vi "Process Dichotomie.vi"(7 "Movable in":refnum<class "Movable.lvclass">, 11 "Collision in":refnum<class "Collision.lvclass">) -> (2 "Coordinates with dichotomie[] out":T1[](array[typedef]), 5 "Dichotomie out":i32=10)   [LabVIEW 2021, in "Collision.lvclass"]
doc: "MIT Licence\nCopyright (c) 2024 David Grollier"
uses:
  Collision.lvclass
  Type Def/Coordinates.ctl
  Game Componants/Game Board Component/Movable/Movable.lvclass
  Game Componants/Game Board/Game Board.lvclass
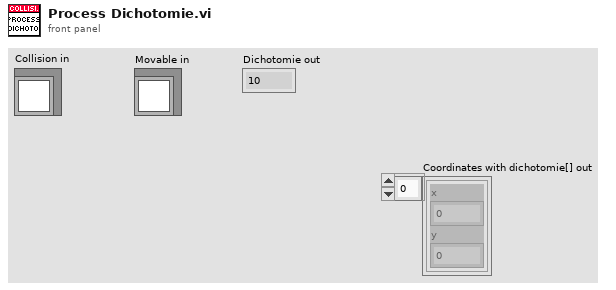
[diagram p1: front panel]
types:
  T1 = typedef "Coordinates.ctl" = cluster{"x":dbl, "y":dbl}
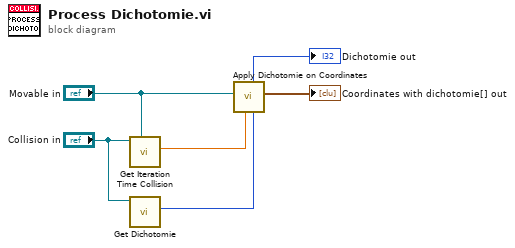
[diagram p0: block diagram]
diagram:
  n1 = call "Get Iteration Time Collision.vi"("Movable in"="Movable in", "Collision in"="Collision in") -> ("Time factor out"=w4:dbl)  [unwired: 9 in]
  n2 = call-dynamic "Get Dichotomie.vi"("Collision in"="Collision in") -> ("Dichotomie out"=w1:i32)  [unwired: 10 in]
  n3 = call "Apply Dichotomie on Coordinates.vi"("Dichotomie in"=w1, "Time factor in"=w4, "Movable in"="Movable in") -> ("Coordinates with dichotomie[]"=→"Coordinates with dichotomie[] out":T1[], "Dichotomie out"=→"Dichotomie out":i32)  [unwired: 7 in]
